vi "Field Emission.vi"(10 "Velocity":dbl, 11 "Pelletron Volts":dbl) -> (3 "Field Emission":ext)   [LabVIEW 2013]
panel:
  # "Field \nEmission=(2*pelletronvolts./v.^2*3e9*4*pi*8.854187817e-12).^3*(3/(4*pi*3200))^2;"
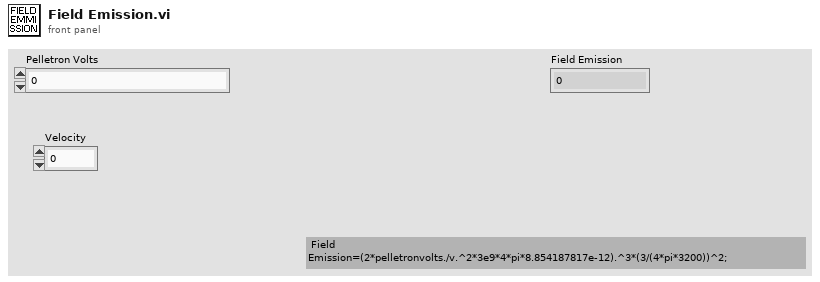
[diagram p1: front panel]
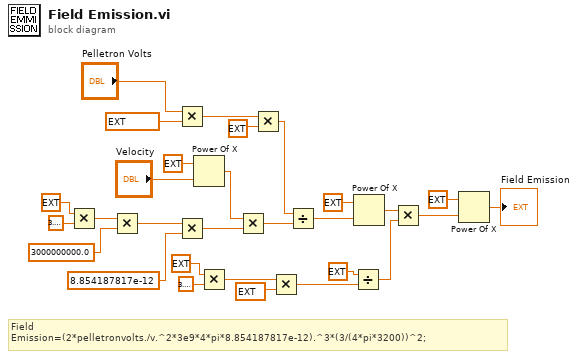
[diagram p0: block diagram]
diagram:
  # "Field \nEmission=(2*pelletronvolts./v.^2*3e9*4*pi*8.854187817e-12).^3*(3/(4*pi*3200))^2;"
  n1 = Multiply(x=ext 4.0, y=3.141592653589793) -> (x*y=w23:ext)
  n2 = Multiply(x=w23, y=3000000000.0) -> (x*y=w21:ext)
  n3 = Multiply(x="Pelletron Volts", y=ext 10000000.0) -> (x*y=w2:ext)
  n4 = Multiply(x=w21, y=8.854187817e-12) -> (x*y=w18:ext)
  n5 = Power Of X(1:"Velocity", 2:ext 2.0 ("y")) -> (0:w19:ext)
  n6 = Multiply(x=ext 4.0 ("y"), y=3.141592653589793) -> (x*y=w6:ext)
  n7 = Multiply(x=w19, y=w18) -> (x*y=w16:ext)
  n8 = Multiply(x=w2, y=ext 2.0) -> (x*y=w28:ext)
  n9 = Multiply(x=w6, y=ext 3200.0) -> (x*y=w4:ext)
  n10 = Divide(x=w28, y=w16) -> (x/y=w15:ext)
  n11 = Divide(x=ext 3.0, y=w4) -> (x/y=w9:ext)
  n12 = Power Of X(1:w15, 2:ext 3.0) -> (0:w14:ext)
  n13 = Multiply(x=w14, y=w9) -> (x*y=w13:ext)
  n14 = Power Of X(1:w13, 2:ext 2.0) -> (0:→"Field Emission":ext)
